vi "CTRE_PigeonIMU_GetStartupStatus.vi"(8 "error in (no error)":errorcluster, 11 "PigeonIMUDevRef":T2={"DeviceStatus"={"status"=FALSE, "code"=0, "source"=""}, "Device Number"=0, "Type"=352321536, "Device ID"=0, "Handle"=0, "UsageFrame"=0, "Library Path"=path ""} {"Type" items=["CAN"=352321536, "TalonSRX"=33554432]}) -> (0 "error out":errorcluster, 2 "Startup Status":T1, 3 "PigeonIMUDevRef":T2={"DeviceStatus"={"status"=FALSE, "code"=0, "source"=""}, "Device Number"=0, "Type"=352321536, "Device ID"=0, "Handle"=0, "UsageFrame"=0, "Library Path"=path ""} {"Type" items=["CAN"=352321536, "TalonSRX"=33554432]})   [LabVIEW 2016]
uses:
  <vilib>/Rock Robotics/WPI/ThirdParty/Sensors/Pigeon IMU/CTRE_PigeonIMU_DeviceRef.ctl
  <vilib>/Rock Robotics/WPI/ThirdParty/Sensors/Pigeon IMU/CTRE_PigeonIMU_ConnectionType.ctl
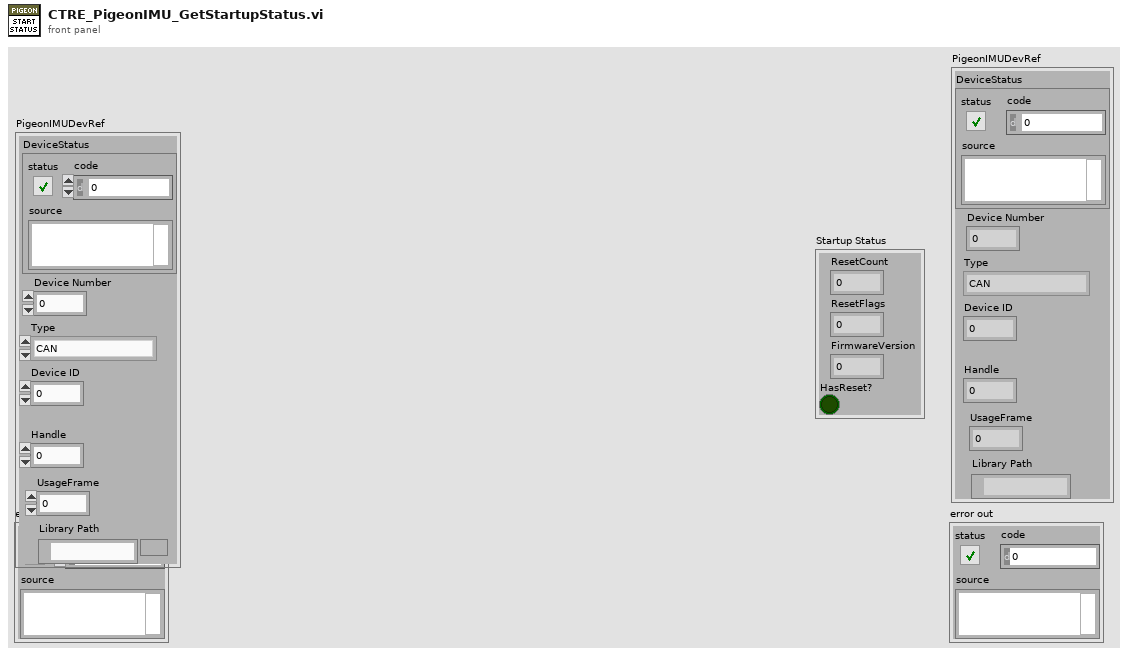
[diagram p1: front panel]
types:
  T1 = cluster{"ResetCount":i32, "ResetFlags":i32, "FirmwareVersion":i32, "HasReset?":bool}
  T2 = typedef "CTRE_PigeonIMU_DeviceRef.ctl" = cluster{"DeviceStatus":errorcluster, "Device Number":u8, "Type":T3, "Device ID":u32, "Handle":u64, "UsageFrame":u32, "Library Path":path}
  T3 = typedef "CTRE_PigeonIMU_ConnectionType.ctl" = u32
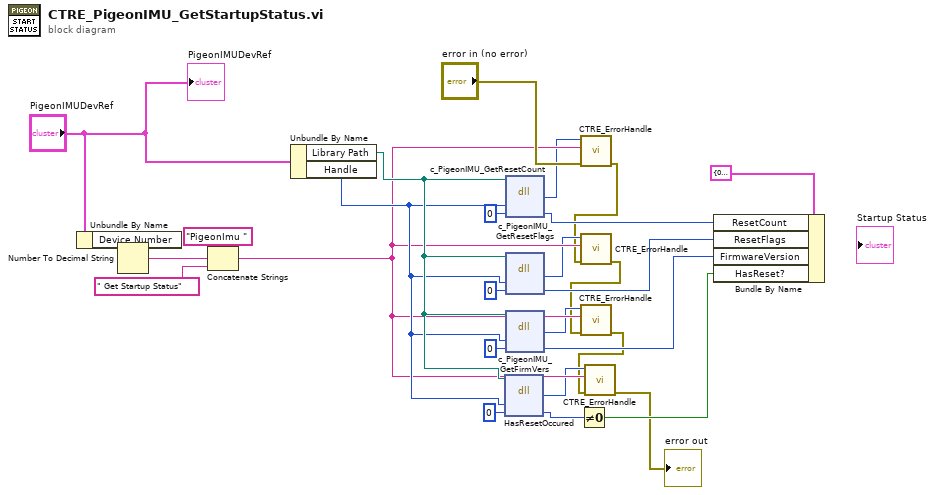
[diagram p0: block diagram]
diagram:
  n1 = Unbundle By Name("PigeonIMUDevRef") -> ("Device Number"=w15:u8)
  n2 = Number To Decimal String(number=w15) -> (decimal integer string=w14:string)  [unwired: 1 in]
  n3 = Concatenate Strings("PigeonImu " ("string"), w14, " Get Startup Status" ("string")) -> (w9:string)
  n4 = Unbundle By Name("PigeonIMUDevRef") -> ("Library Path"=w19:path, "Handle"=w18:u64)
  n5 = dll-call lib="?" fn="HasResetOccured"(path in=w19, "handle"=w18, "value"=0) -> ("return type"=w5:i32, "value"=w17:u8)  [unwired: 3 in, 2 out]
  n6 = dll-call lib="?" fn="c_PigeonIMU_GetResetCount"(path in=w19, "handle"=w18, "value"=0) -> ("return type"=w8:i32, "value"=w27:i32)  [unwired: 3 in, 2 out]
  n7 = dll-call lib="?" fn="c_PigeonIMU_GetResetFlags"(path in=w19, "handle"=w18, "value"=0) -> ("return type"=w7:i32, "value"=w26:i32)  [unwired: 3 in, 2 out]
  n8 = dll-call lib="?" fn="c_PigeonIMU_GetFirmVers"(path in=w19, "handle"=w18, "value"=0) -> ("return type"=w6:i32, "value"=w25:i32)  [unwired: 3 in, 2 out]
  n9 = Not Equal To 0?(x=w17) -> (x != 0?=w16:bool)
  n10 = call <vilib>:"CTRE_ErrorHandle.vi"("error in"="error in (no error)", "origin"=w9, "code"=w8) -> ("error out"=w4:errorcluster)  [unwired: 8 in]
  n11 = call <vilib>:"CTRE_ErrorHandle.vi"("error in"=w4, "origin"=w9, "code"=w7) -> ("error out"=w3:errorcluster)  [unwired: 8 in]
  n12 = call <vilib>:"CTRE_ErrorHandle.vi"("error in"=w3, "origin"=w9, "code"=w6) -> ("error out"=w2:errorcluster)  [unwired: 8 in]
  n13 = call <vilib>:"CTRE_ErrorHandle.vi"("error in"=w2, "origin"=w9, "code"=w5) -> ("error out"=→"error out":errorcluster)  [unwired: 8 in]
  n14 = Bundle By Name(cluster=T1 {"ResetCount"=0, "ResetFlags"=0, "FirmwareVersion"=0, "HasReset?"=FALSE} ("StartupStatus"), "ResetCount"=w27, "ResetFlags"=w26, "FirmwareVersion"=w25, "HasReset?"=w16) -> ()  [unwired: 1 out]
  "PigeonIMUDevRef" <- "PigeonIMUDevRef"
